vi "ControllerMain.vi"(8 "Error In":errorcluster, 11 "Control Mode":T4(ring)) -> (0 "Error Out":errorcluster, 3 "Robot Inputs":T3, 4 "Joystick1DevRef":T1={"Device"=enum."USB 1"}, 5 "Stick0 Buttons":bool[](array[boolean]), 6 "Joystick0DevRef":T1={"Device"=enum."USB 1"}, 7 "Stick0 Axes":dbl[](array[numeric]))   [LabVIEW 2017]
uses:
  TeleopCommands.ctl
  <vilib>/Rock Robotics/WPI/Joystick/WPI_JoystickDevRef.ctl
  <vilib>/Rock Robotics/WPI/Joystick/WPI_JoystickDeviceEnum.ctl
  <vilib>/Rock Robotics/WPI/Utilities/WPI_GetSetVariantRefNum.vi
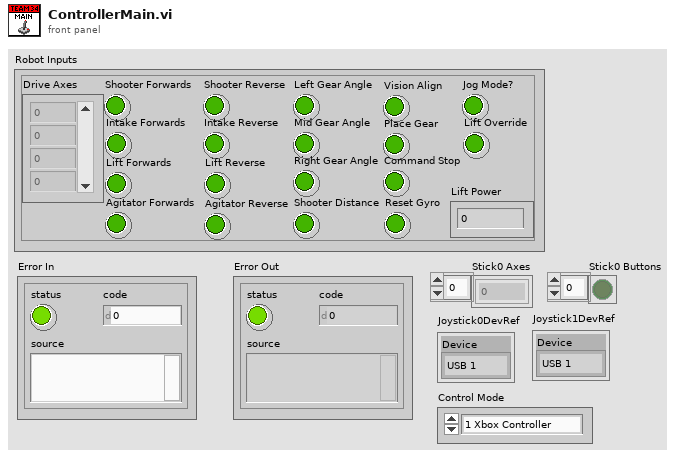
[diagram p1: front panel]
types:
  T1 = typedef "WPI_JoystickDevRef.ctl" = cluster{"Device":T2}
  T2 = typedef "WPI_JoystickDeviceEnum.ctl" = enum16{"USB 0", "USB 1", "USB 2", "USB 3", "USB 4", "USB 5"}
  T3 = typedef "TeleopCommands.ctl" = cluster{"Drive Axes":dbl[], "Shooter Forwards":bool, "Shooter Reverse":bool, "Intake Forwards":bool, "Intake Reverse":bool, "Lift Forwards":bool, "Lift Reverse":bool, "Agitator Forwards":bool, "Agitator Reverse":bool, "Left Gear Angle":bool, "Mid Gear Angle":bool, "Right Gear Angle":bool, "Shooter Distance":bool, "Vision Align":bool, "Place Gear":bool, "Command Stop":bool, "Reset Gyro":bool, "Jog Mode?":bool, "Lift Override":bool, "Lift Power":dbl}
  T4 = enum16{"1 Xbox Controller", "2 Xbox Controllers"}
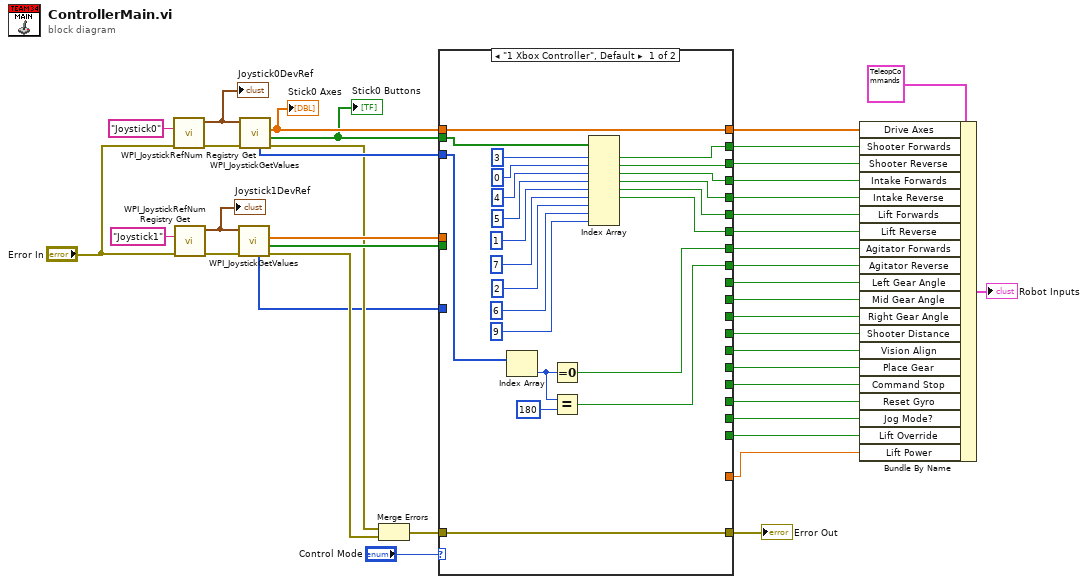
[diagram p0: block diagram]
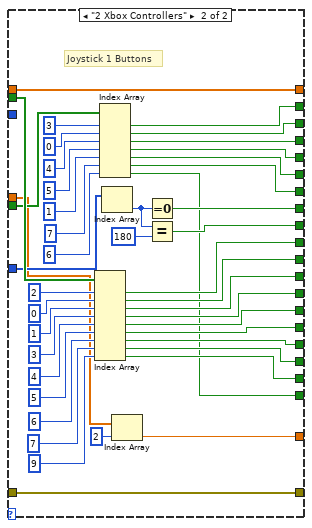
[diagram p2: hidden frame]
diagram:
  n1 = call <vilib>:"WPI_JoystickRefNum Registry Get.vi"("error in (no error)"="Error In", "refnum name"="Joystick0") -> ("error out"=w35:errorcluster, "JoystickDevRef"=w40:T1)  [unwired: 8 out]
  "Joystick0DevRef" <- w40
  n2 = call <vilib>:"WPI_JoystickRefNum Registry Get.vi"("error in (no error)"="Error In", "refnum name"="Joystick1") -> ("error out"=w36:errorcluster, "JoystickDevRef"=w37:T1)  [unwired: 8 out]
  "Joystick1DevRef" <- w37
  n3 = call <vilib>:"WPI_JoystickGetValues.vi"("error in (no error)"=w36, "JoystickDevRef"=w37) -> ("error out"=w17:errorcluster, "Buttons"=w31:bool[], "Axes"=w30:dbl[], "POVs"=w14:i16[])  [unwired: 5 in, 1 out]
  n4 = call <vilib>:"WPI_JoystickGetValues.vi"("error in (no error)"=w35, "JoystickDevRef"=w40) -> ("error out"=w18:errorcluster, "Buttons"=w32:bool[], "Axes"=w33:dbl[], "POVs"=w20:i16[])  [unwired: 5 in, 1 out]
  "Stick0 Axes" <- w33
  "Stick0 Buttons" <- w32
  n5 = Merge Errors(w18, w17) -> (w16:errorcluster)
  n6 = case shown="\"1 Xbox Controller\", Default" "Control Mode" {
    tunnel: w33 -> [w63 w107]
    tunnel: w32 -> [w62 w106]
    tunnel: w31 -> [_ w104]
    tunnel: w30 -> [_ w66]
    tunnel: [w63 w107] -> w29
    tunnel: [w55 w93] -> w28
    tunnel: [w54 w92] -> w27
    tunnel: [w53 w100] -> w26
    tunnel: [w52 w98] -> w25
    tunnel: [w51 w96] -> w24
    tunnel: [w50 w95] -> w23
    tunnel: [w46 w88] -> w22
    tunnel: [w43 w87] -> w21
    tunnel: w20 -> [w47 _]
    tunnel: [w42 w105] -> w15
    tunnel: w16 -> [w42 w105]
    tunnel: w14 -> [_ w89]
    tunnel: [_ w82] -> w13
    tunnel: [_ w81] -> w12
    tunnel: [_ w80] -> w11
    tunnel: [_ w79] -> w10
    tunnel: [_ w78] -> w9
    tunnel: [_ w77] -> w8
    tunnel: [_ w73] -> w7
    tunnel: [_ w71] -> w6
    tunnel: [_ w69] -> w5
    tunnel: [_ w67] -> w4
    tunnel: [_ w64] -> w1
    frame "1 Xbox Controller", Default {
      n7 = Index Array(array=w47) -> (element=w45:i16)  [unwired: 1 in]
      n8 = Equal To 0?(x=w45) -> (x = 0?=w46:bool)
      n9 = Equal?(x=w45, y=i16 180) -> (x = y?=w43:bool)
      n10 = Index Array(array=w62, index #1=3 ("index"), index #2=0 ("index"), index #3=4 ("index"), index #4=5 ("index"), index #5=1 ("index"), index #6=7 ("index"), index #7=2 ("index"), index #8=6 ("index"), index #9=9 ("index")) -> (element #1=w55:bool, element #2=w54:bool, element #3=w53:bool, element #4=w52:bool, element #5=w51:bool, element #6=w50:bool)  [unwired: 3 out]
    }
    frame "2 Xbox Controllers" {
      # "Joystick 1 Buttons"
      n11 = Index Array(array=w106, index #1=2 ("index"), index #2=0 ("index"), index #3=1 ("index"), index #4=3 ("index"), index #5=4 ("index"), index #6=5 ("index"), index #7=6 ("index"), index #8=7 ("index"), index #9=9 ("index")) -> (element #1=w82:bool, element #2=w81:bool, element #3=w80:bool, element #4=w79:bool, element #5=w78:bool, element #6=w77:bool, element #7=w73:bool, element #8=w71:bool, element #9=w69:bool)
      n12 = Index Array(array=w104, index #1=3 ("index"), index #2=0 ("index"), index #3=4 ("index"), index #4=5 ("index"), index #5=1 ("index"), index #6=7 ("index"), index #7=6 ("index")) -> (element #1=w93:bool, element #2=w92:bool, element #3=w100:bool, element #4=w98:bool, element #5=w96:bool, element #6=w95:bool, element #7=w67:bool)
      n13 = Index Array(array=w89) -> (element=w91:i16)  [unwired: 1 in]
      n14 = Index Array(array=w66, index=2) -> (element=w64:dbl)
      n15 = Equal To 0?(x=w91) -> (x = 0?=w88:bool)
      n16 = Equal?(x=w91, y=i16 180) -> (x = y?=w87:bool)
    }
  }
  "Error Out" <- w15
  n17 = Bundle By Name(cluster=T3 {"Drive Axes"=[], "Shooter Forwards"=FALSE, "Shooter Reverse"=FALSE, "Intake Forwards"=FALSE, "Intake Reverse"=FALSE, "Lift Forwards"=FALSE, "Lift Reverse"=FALSE, "Agitator Forwards"=FALSE, "Agitator Reverse"=FALSE, "Left Gear Angle"=FALSE, "Mid Gear Angle"=FALSE, "Right Gear Angle"=FALSE, "Shooter Distance"=FALSE, "Vision Align"=FALSE, "Place Gear"=FALSE, "Command Stop"=FALSE, "Reset Gyro"=FALSE, "Jog Mode?"=FALSE, "Lift Override"=FALSE, "Lift Power"=0.0} ("Robot Inputs"), "Drive Axes"=w29, "Shooter Forwards"=w28, "Shooter Reverse"=w27, "Intake Forwards"=w26, "Intake Reverse"=w25, "Lift Forwards"=w24, "Lift Reverse"=w23, "Agitator Forwards"=w22, "Agitator Reverse"=w21, "Left Gear Angle"=w13, "Mid Gear Angle"=w12, "Right Gear Angle"=w11, "Shooter Distance"=w10, "Vision Align"=w9, "Place Gear"=w8, "Command Stop"=w7, "Reset Gyro"=w6, "Jog Mode?"=w5, "Lift Override"=w4, "Lift Power"=w1) -> (→"Robot Inputs":T3)
